vi "ReadPressure Example.vi"() -> ()   [LabVIEW 2019]
uses:
  BrooksDLL.dll
panel:
  out "S2 String":string
  out "S1 String":string
  out "S2":u8 format="%.0x"
  out "S1":u8 format="%.0x"
  out "Function Output Comment":string
  out "Pressure Unit String":string
  out "Pressure Unit Code":u8
  out "Pressure":sgl format="%.2f"
  out "output param":i32
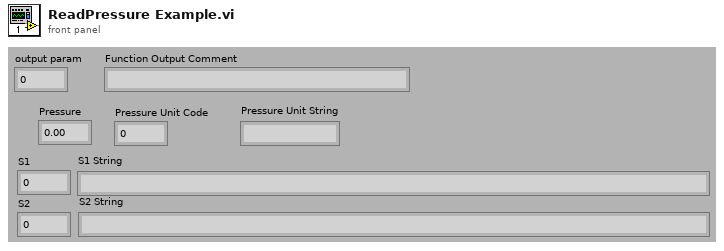
[diagram p1: front panel]
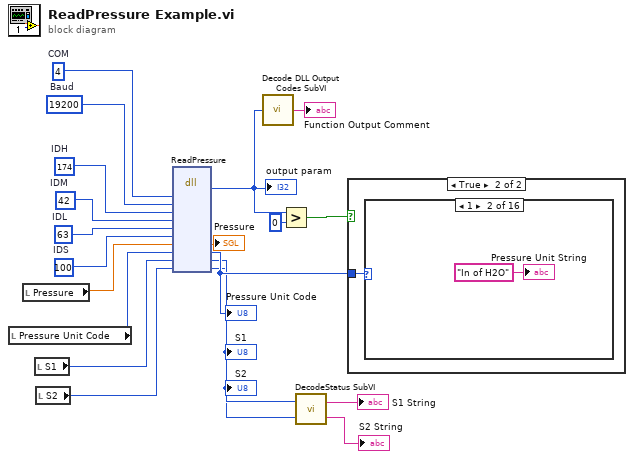
[diagram p0: block diagram]
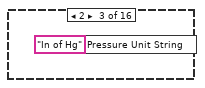
[diagram p4: hidden frame]
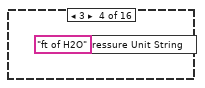
[diagram p5: hidden frame]
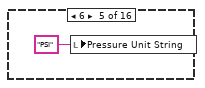
[diagram p6: hidden frame]
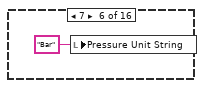
[diagram p7: hidden frame]
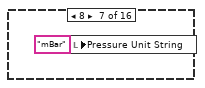
[diagram p8: hidden frame]
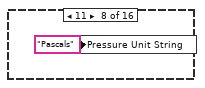
[diagram p9: hidden frame]
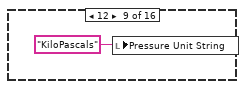
[diagram p10: hidden frame]
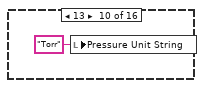
[diagram p11: hidden frame]
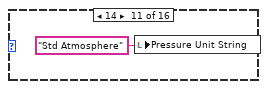
[diagram p12: hidden frame]
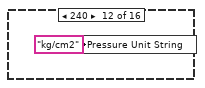
[diagram p13: hidden frame]
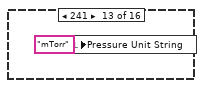
[diagram p14: hidden frame]
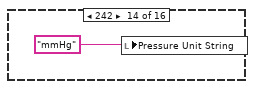
[diagram p15: hidden frame]
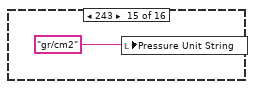
[diagram p16: hidden frame]
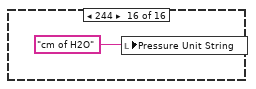
[diagram p17: hidden frame]
diagram:
  w15 = u8 100  # IDS
  w16 = u8 63  # IDL
  w17 = u8 42  # IDM
  w18 = u8 174  # IDH
  w19 = 19200  # Baud
  w20 = 4  # COM
  n1 = local read "Pressure Unit Code"() -> (w10:u8)
  n2 = local read "Pressure"() -> (w7:sgl)
  n3 = local read "S1"() -> (w6:u8)
  n4 = local read "S2"() -> (w5:u8)
  n5 = dll-call lib="G:/Developpement_de_Programmes/Programmes/Controle de pression/164J027_AD/Brooks DLL 1.0.1.0 32bit/Brooks DLL 1.0.1.0 Release 10032016/S Protocol/BrooksDLL.dll" fn="ReadPressure"("COM"=w20, "Baud"=w19, "IDH"=w18, "IDM"=w17, "IDL"=w16, "IDS"=w15, "Pressure"=w7, "PressureUnitCoce"=w10, "S1"=w6, "S2"=w5) -> (w12:i32, "Pressure"=→"Pressure":sgl, "PressureUnitCoce"=w9:u8, "S1"=w4:u8, "S2"=w3:u8)  [unwired: 9 in, 2 out]
  "output param" <- w12
  "Pressure Unit Code" <- w9
  "S1" <- w4
  "S2" <- w3
  n6 = call "Decode DLL Output Codes SubVI.vi"("Numeric"=w12) -> ("Function Output Comment"=→"Function Output Comment":string)
  n7 = Greater?(x=w12, y=0) -> (0:w14:bool)
  n8 = call "DecodeStatus SubVI.vi"("S2"=w3, "S1"=w4) -> ("S2 String"=→"S2 String":string, "S1 String"=→"S1 String":string)
  n9 = case shown="True" w14 {
    tunnel: w9 -> [_ w21]
    frame False {
    }
    frame True {
      n10 = case shown="1" w21 {
        frame 0, Default {
        }
        frame 1 {
          "Pressure Unit String" <- "In of H2O"
        }
        frame 2 {
          n11 = local write "Pressure Unit String"("In of Hg") -> ()
        }
        frame 3 {
          n12 = local write "Pressure Unit String"("ft of H2O") -> ()
        }
        frame 6 {
          n13 = local write "Pressure Unit String"("PSI") -> ()
        }
        frame 7 {
          n14 = local write "Pressure Unit String"("Bar") -> ()
        }
        frame 8 {
          n15 = local write "Pressure Unit String"("mBar") -> ()
        }
        frame 11 {
          n16 = local write "Pressure Unit String"("Pascals") -> ()
        }
        frame 12 {
          n17 = local write "Pressure Unit String"("KiloPascals") -> ()
        }
        frame 13 {
          n18 = local write "Pressure Unit String"("Torr") -> ()
        }
        frame 14 {
          n19 = local write "Pressure Unit String"("Std Atmosphere") -> ()
        }
        frame 240 {
          n20 = local write "Pressure Unit String"("kg/cm2") -> ()
        }
        frame 241 {
          n21 = local write "Pressure Unit String"("mTorr") -> ()
        }
        frame 242 {
          n22 = local write "Pressure Unit String"("mmHg") -> ()
        }
        frame 243 {
          n23 = local write "Pressure Unit String"("gr/cm2") -> ()
        }
        frame 244 {
          n24 = local write "Pressure Unit String"("cm of H2O") -> ()
        }
      }
    }
  }
